vi "diffraction pattern v1.6.vi"() -> ()   [LabVIEW 2019]
panel:
  in  "Save":bool
  in  "hold":bool
  out "Current Flux":dbl=5.0
  out "Remaining steps":i32
  in  "Exit":bool
  in  "Run":bool
  out "Help":string="1. before run, set the paramaters on the left of the screen.\n2. flux (magnetic field) is in unit of flux quanta.\n3. Phaserange is in the unit of Pi, the CPR will be build up according to phase range of [-Phaserange/2,Phaserang/2], and such CPR will be  a periodic function with Phaserange as period. Enter integer number  of multiple times of 4 is preferred.\n4. Use the step setting tab to set resolution of the calculation, you can set how many points is used to define the width of the Josephson junction, how many points to represent the Phaserange\n5. Then you can choose which type of the CPR is used.\n6. Depending on the choose of the CPR, you may want to set the strength of the MBS, \"a\" parameter, the width of the gaussian function used, and the pattern of parity of MBS. Parity pattern has to have same number of elements for positive and negative range.\nEnter the parity 1 or -1 for positive and negative phase +-Pi, +-3Pi, +-5Pi etc.. in to the two arrays.\n7. You can use the index control to read the array elements, then enter the value, you can also delete an element of array by right click, the number of array elements is not limited.\n8. You can change the x,y range, zoom, create cursor etc. to help analyse the plot. Right click to save the data into excel.\n\nEnjoy!\nGuang Yue\n\n\n"
  in  "parity for negative phase":i32[](array[numeric])=[1, -1, -1, 1]
  in  "Strenth of MBS":dbl=0.5
  in  "parity for positive phase":i32[](array[numeric])=[1, -1, 1, 1]
  in  "Gaussian width":dbl=0.2
  in  "Tab Control":enum32{"Range", "Steps setting"}(tab)
  in  "flux start":dbl=-5.0
  in  "flux end":dbl=5.0
  in  "flux step":dbl=0.1
  in  "phaserange in Pi":i32=16
  in  "Geometry":i32=201
  in  "Phase steps":i32=201
  in  "CPR Type":T1(ring)
  out "Total time s":dbl=5.020437899999706
  in  "stop loop":bool
  out "Diffraction pattern plot":cluster{cluster{dbl, "icn":dbl}[]}[](graph)
  out "Ic negative":dbl=-0.0009989221220817583
  out "Ic positive":dbl=0.000998922122081775
  out "error out":errorcluster
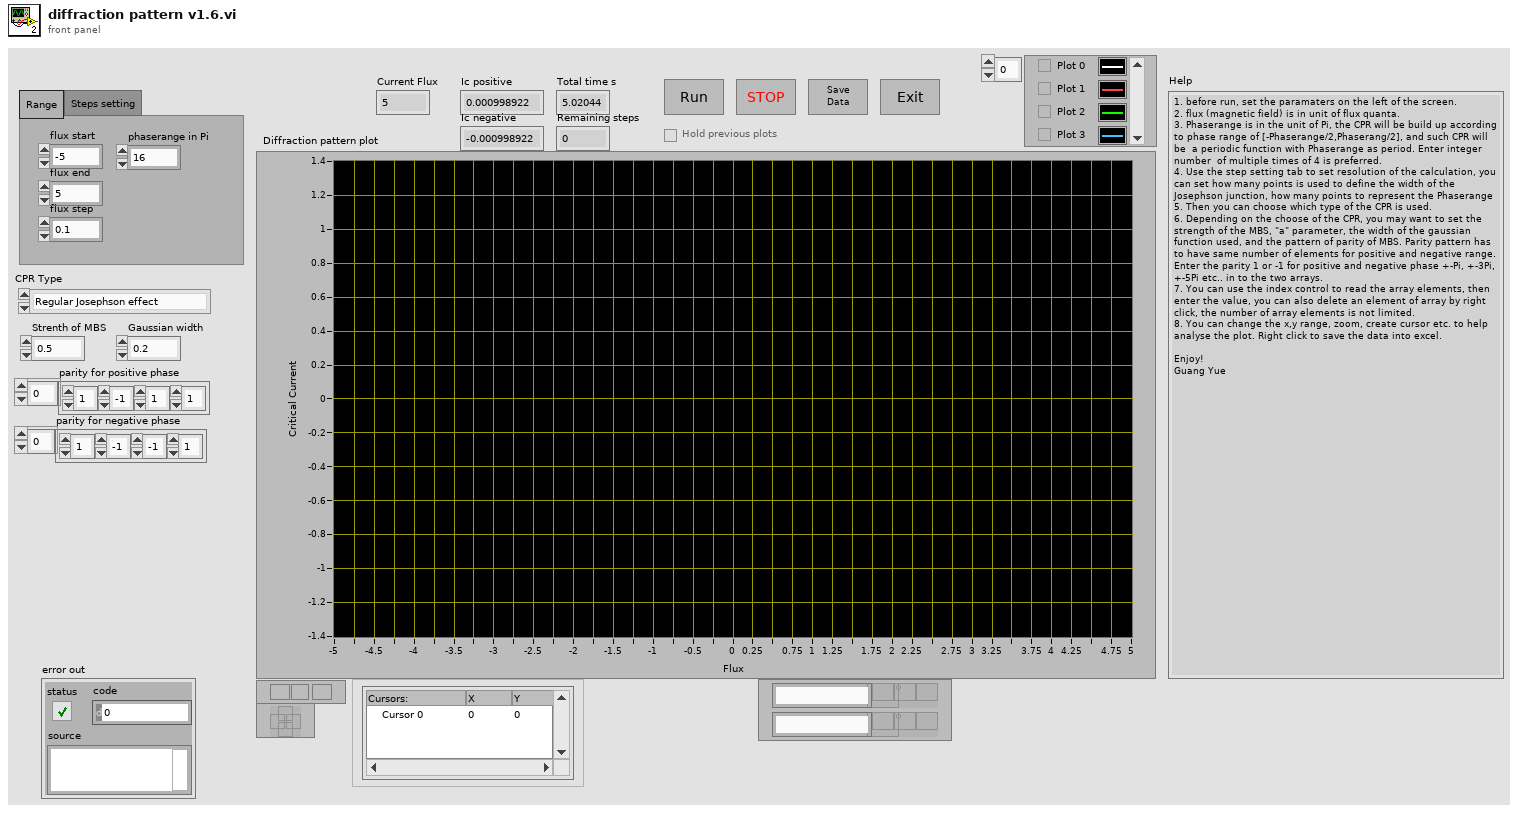
[diagram p1: front panel]
types:
  T1 = enum16{"Regular Josephson effect", "Non-local MBS", "Local MBS same parity", "Local MBS different parity"}
  T2 = enum32{"invalid app kind", "Development System", "Run Time System", "Student Edition", "Embedded LabVIEW", "Evaluation", "Custom"}
  T3 = enum8{"Enabled", "Disabled", "Disabled and Grayed Out"}
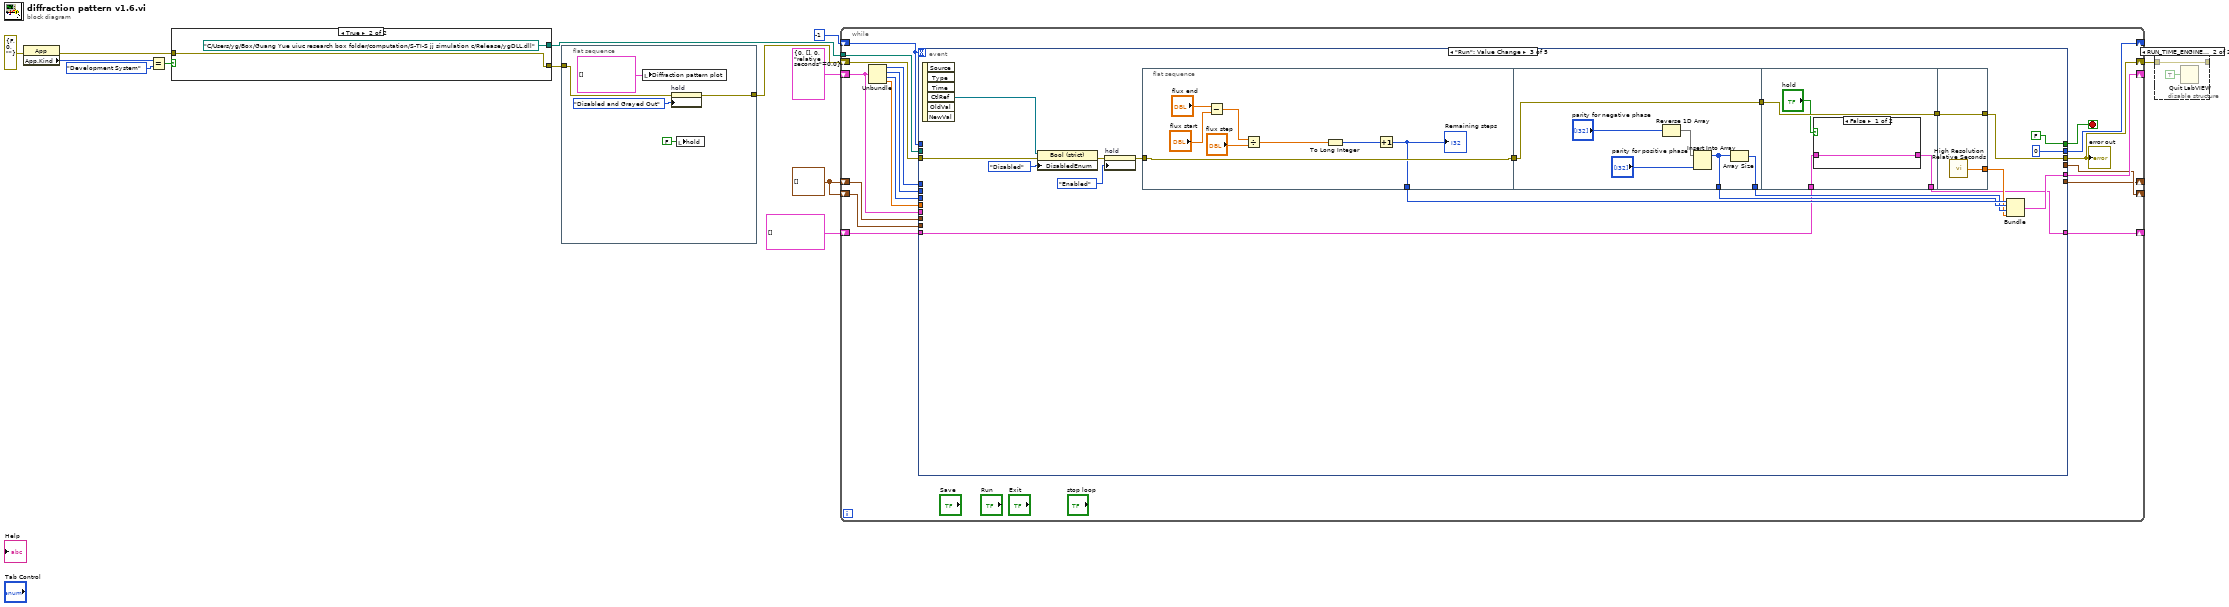
[diagram p0: block diagram]
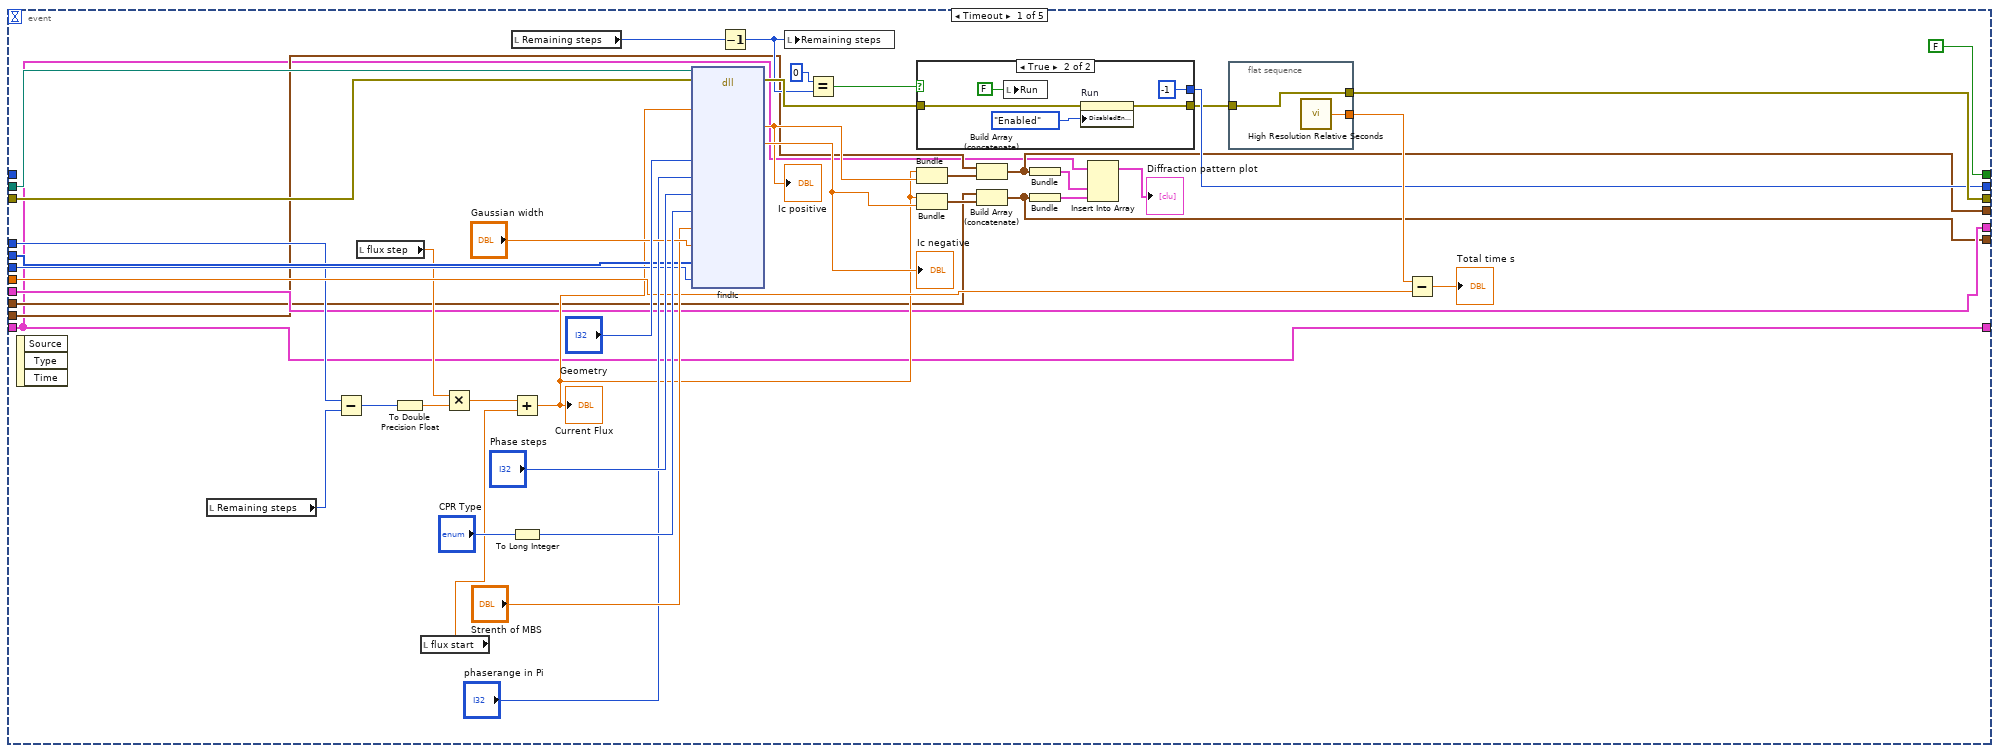
[diagram p3: hidden frame]
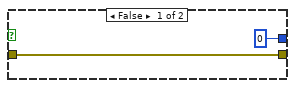
[diagram p4: hidden frame]
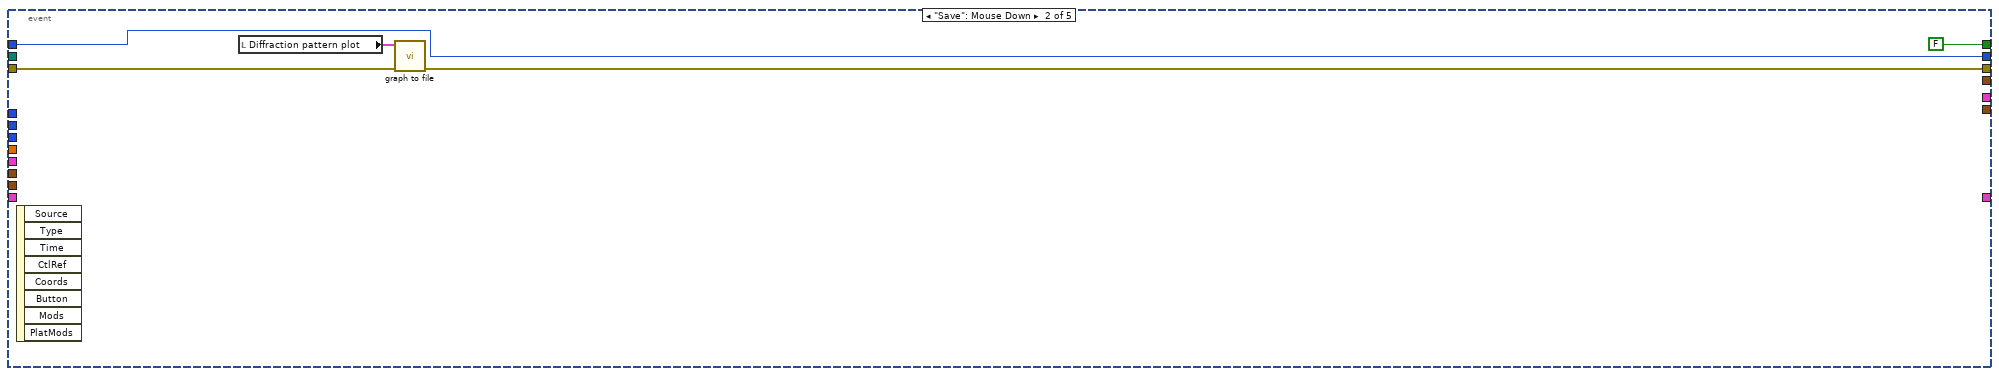
[diagram p5: hidden frame]
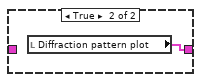
[diagram p6: hidden frame]
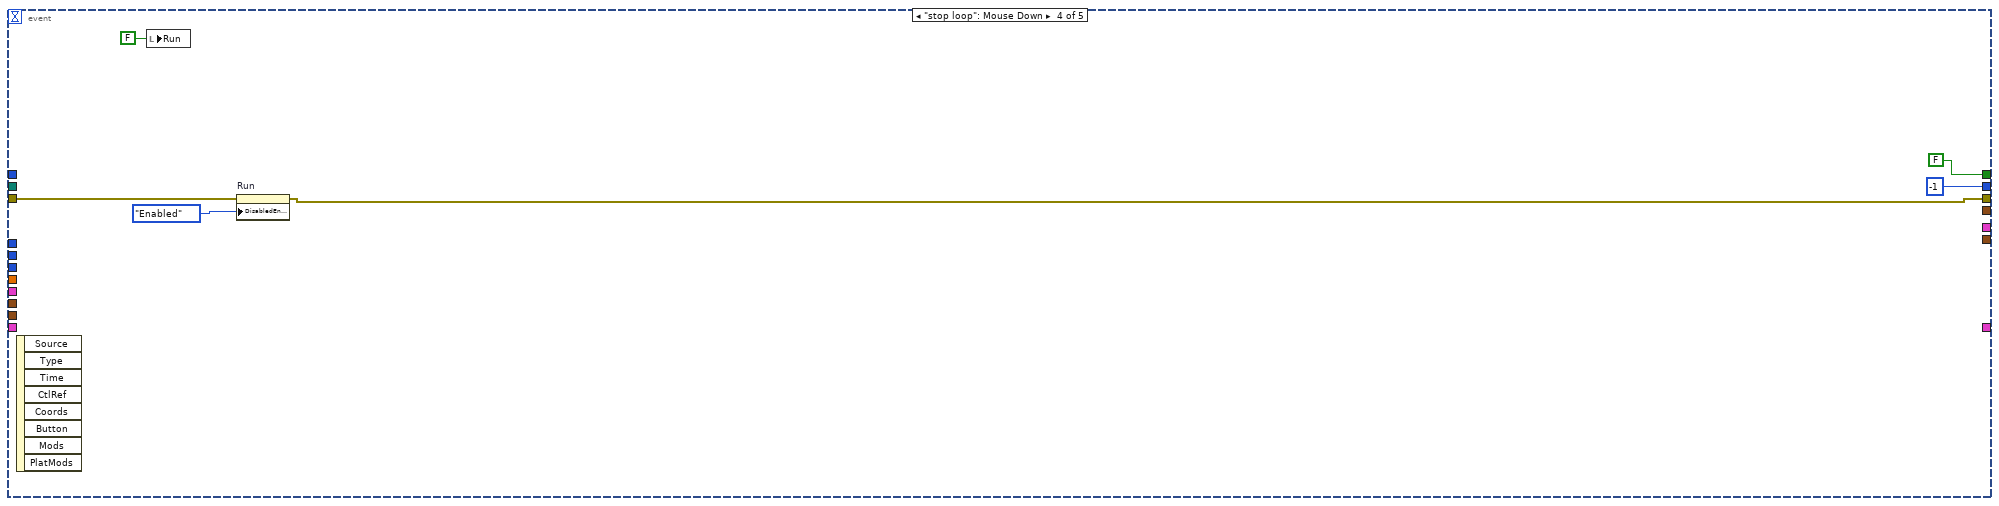
[diagram p7: hidden frame]
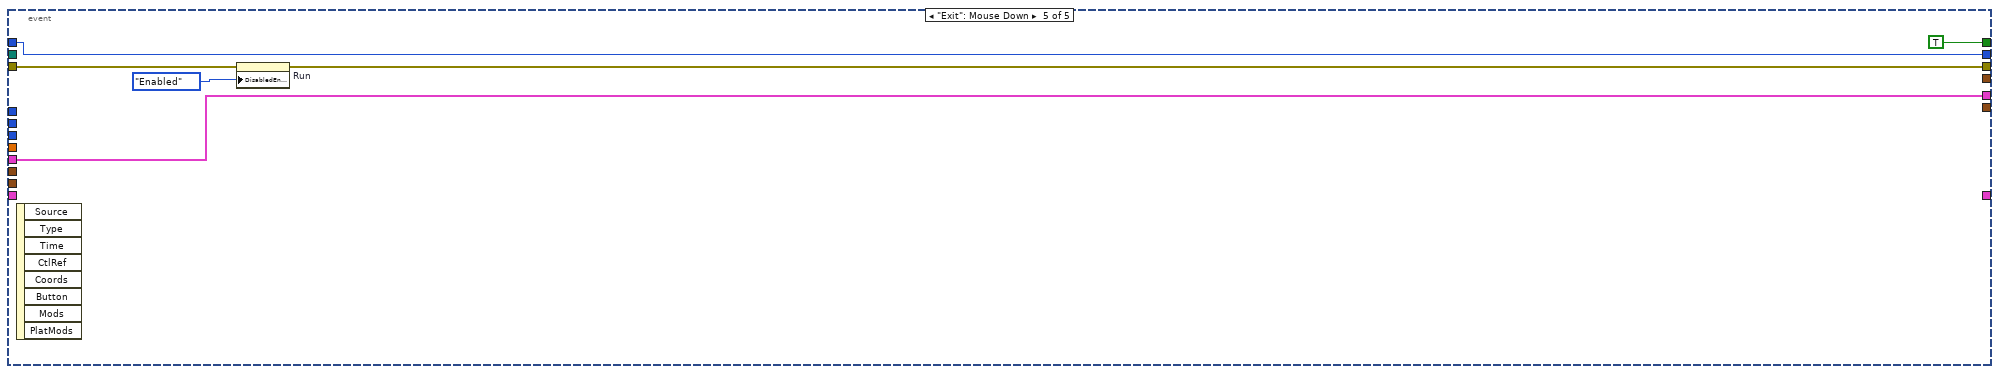
[diagram p8: hidden frame]
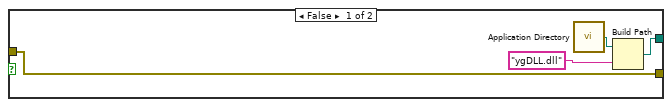
[diagram p9: hidden frame]
diagram:
  w5 = cluster{dbl, "inp":dbl}[] []
  n1 = property class="App"(error in=errorcluster {"status"=FALSE, "code"=0, "source"=""} ("error out")) -> (error out=w9:errorcluster, "App.Kind"=w12:T2)  [unwired: 1 in, 1 out]
  n2 = Equal?(x=w12, y=T2."Development System" ("Application:Kind")) -> (x = y?=w10:bool)
  n3 = case shown="True" w10 {
    tunnel: [w15 path "C:/Users/yg/Box/Guang Yue uiuc research box folder/computation/S-TI-S jj simulation c/Release/ygDLL.dll"] -> w8
    tunnel: w9 -> [w14 w18]
    tunnel: [w14 w18] -> w2
    frame False {
      n4 = call <vilib>:"Application Directory.vi"() -> ("Application Directory"=w17:path)
      n5 = Build Path(base path=w17, name or relative path="ygDLL.dll") -> (appended path=w15:path)
    }
    frame True {
    }
  }
  n6 = flat-sequence {
    tunnel: w2 -> [w23]
    tunnel: [w22] -> w1
    frame #0 {
      n7 = local write "Diffraction pattern plot"(cluster{cluster{dbl, "icn":dbl}[]}[] [] ("appended array")) -> ()
      n8 = property on="hold" class="Bool (strict)"(error in=w23, "DisabledEnum"=T3."Disabled and Grayed Out" ("Disabled")) -> (error out=w22:errorcluster)  [unwired: 1 in, 1 out]
      n9 = local write "hold"(FALSE ("hold")) -> ()
    }
  }
  n10 = while {
    tunnel: w8 -> [w39]
    shift-right: [w41] -> _
    shift-left: -1 -> [w32]
    shift-right: [w42] -> _
    shift-left: cluster{i32, i32[], i32, "relative seconds":dbl} {0, [], 0, "relative seconds"=0.0} -> [w33]
    shift-right: [w35] -> w4
    shift-left: w1 -> [w40]
    shift-right: [w30] -> _
    shift-left: w5 -> [w31]
    shift-right: [w29] -> _
    shift-left: w5 -> [w28]
    shift-right: [w25] -> _
    shift-left: cluster{cluster{dbl, "icn":dbl}[]}[] [] ("appended array") -> [w26]
    stop <- w27 stop-if-true
    n11 = Unbundle(w33) -> (w34:i32, w38:i32[], w37:i32, "relative seconds"=w36:dbl)
    n12 = event shown="[2] \"Run\": Value Change" {
      selector: _ -> [_ _ _ _ _]
      dyn-events: _ -> [_ _ _ _ _]
      timeout: w32 -> [_ _ _ _ _]
      tunnel: [w53 _ w112 _ w152] -> w42
      tunnel: [w55 w99 0 -1 w153] -> w41
      tunnel: w40 -> [w72 w98 w110 w146 w150]
      tunnel: w39 -> [w71 _ _ _ _]
      tunnel: w38 -> [w70 _ _ _ _]
      tunnel: w37 -> [w69 _ _ _ _]
      tunnel: w36 -> [w68 _ _ _ _]
      tunnel: [w67 w96 w109 w144 w148] -> w35
      tunnel: w34 -> [w66 _ _ _ _]
      tunnel: w33 -> [w53 _ _ _ w152]
      tunnel: w32 -> [_ w99 _ _ w153]
      tunnel: w31 -> [w50 _ _ _ _]
      tunnel: [w51 _ _ _ _] -> w30
      tunnel: [w49 _ _ _ _] -> w29
      tunnel: w28 -> [w48 _ _ _ _]
      tunnel: [FALSE FALSE FALSE FALSE TRUE] -> w27
      tunnel: w26 -> [w43 _ w104 _ _]
      tunnel: [w43 _ w105 _ _] -> w25
      event Timeout {
        n13 = event-data() -> ()  [unwired: 1 in, 3 out]
        n14 = local read "Remaining steps"() -> (w65:i32)
        n15 = Subtract(x=w66, y=w65) -> (x-y=w63:i32)
        n16 = local read "flux step"() -> (w64:dbl)
        n17 = To Double Precision Float(number=w63) -> (double precision float=w81:dbl)
        n18 = local read "flux start"() -> (w62:dbl)
        n19 = Multiply(x=w64, y=w81) -> (x*y=w82:dbl)
        n20 = local read "Remaining steps"() -> (w59:i32)
        n21 = Add(x=w82, y=w62) -> (x+y=w61:dbl)
        "Current Flux" <- w61
        n22 = To Long Integer(number="CPR Type") -> (32bit integer=w86:i32)
        n23 = dll-call lib="C:/Users/yg/Box/Guang Yue uiuc research box folder/computation/S-TI-S jj simulation c/Release/ygDLL.dll" fn="findIc"(path in=w71, error in=w72, "flux"=w61, "nw"="Geometry", "phaserange"="phaserange in Pi", "nphase"="Phase steps", "cpr"=w86, "a"="Strenth of MBS", "gw"="Gaussian width", "parity"=w70, "parity_l"=w69) -> (error out=w60:errorcluster, "inp"=w83:dbl, "icn"=w84:dbl)  [unwired: 13 in, 1 out]
        "Ic positive" <- w83
        "Ic negative" <- w84
        n24 = Decrement(x=w59) -> (x-1=w57:i32)
        n25 = local write "Remaining steps"(w57) -> ()
        n26 = Equal?(x=0, y=w57) -> (x = y?=w56:bool)
        n27 = case shown="True" w56 {
          tunnel: w60 -> [w87 w92]
          tunnel: [0 -1] -> w55
          tunnel: [w87 w91] -> w54
          frame False {
          }
          frame True {
            n28 = local write "Run"(FALSE ("Run")) -> ()
            n29 = property on="Run" class="Bool (strict)"(error in=w92, "DisabledEnum"=T3."Enabled" ("Disabled")) -> (error out=w91:errorcluster)  [unwired: 1 in, 1 out]
          }
        }
        n30 = Bundle(w61, "inp"=w83) -> (w52:cluster{dbl, "inp":dbl})  [unwired: 1 in]
        n31 = Bundle(w61, "icn"=w84) -> (w85:cluster{dbl, "icn":dbl})  [unwired: 1 in]
        n32 = Build Array (concatenate)(w50, w52) -> (w51:cluster{dbl, "inp":dbl}[])
        n33 = Build Array (concatenate)(w48, w85) -> (w49:cluster{dbl, "icn":dbl}[])
        n34 = Bundle(w51) -> (w46:cluster{cluster{dbl, "inp":dbl}[]})  [unwired: 1 in]
        n35 = Bundle(w49) -> (w45:cluster{cluster{dbl, "icn":dbl}[]})  [unwired: 1 in]
        n36 = Insert Into Array(array=w43, new element #1=w46, new element #2=w45) -> (→"Diffraction pattern plot":cluster{cluster{dbl, "icn":dbl}[]}[])  [unwired: 1 in]
        n37 = flat-sequence {
          tunnel: w54 -> [w95]
          tunnel: [w95] -> w67
          tunnel: [w94] -> w80
          frame #0 {
            n38 = call <vilib>:"High Resolution Relative Seconds.vi"() -> ("relative seconds"=w94:dbl)
          }
        }
        n39 = Subtract(x=w80, y=w68) -> (x-y=→"Total time s":dbl)
      }
      event "Save": Mouse Down {
        n40 = event-data() -> ()  [unwired: 1 in, 8 out]
        n41 = local read "Diffraction pattern plot"() -> (w97:cluster{cluster{dbl, "icn":dbl}[]}[])
        n42 = call "graph to file.vi"("error in (no error)"=w98, "Input array"=w97) -> ("error out"=w96:errorcluster)  [unwired: 9 in]
      }
      event "Run": Value Change {
        n43 = event-data() -> ("CtlRef"=w119:refnum<vi>)  [unwired: 1 in, 5 out]
        n44 = property class="Bool (strict)"(reference=w119, error in=w110, "DisabledEnum"=T3."Disabled" ("Disabled")) -> (error out=w103:errorcluster)  [unwired: 1 out]
        n45 = property on="hold" class="Bool (strict)"(error in=w103, "DisabledEnum"=T3."Enabled" ("Disabled")) -> (error out=w102:errorcluster)  [unwired: 1 in, 1 out]
        n46 = flat-sequence {
          tunnel: w102 -> [w121]
          tunnel: [w120] -> w116
          tunnel: [w121] -> w117
          tunnel: w117 -> [w133]
          tunnel: [w129] -> w114
          tunnel: [w128] -> w115
          tunnel: [w133] -> w107
          tunnel: w107 -> [w137]
          tunnel: [w137] -> w106
          tunnel: [w135] -> w105
          tunnel: w104 -> [w134]
          tunnel: [w141] -> w109
          tunnel: w106 -> [w141]
          tunnel: [w140] -> w113
          frame #0 {
            n47 = Subtract(x="flux end", y="flux start") -> (x-y=w126:dbl)
            n48 = Divide(x=w126, y="flux step") -> (x/y=w125:dbl)
            n49 = To Long Integer(number=w125) -> (32bit integer=w124:i32)
            n50 = Increment(x=w124) -> (x+1=w120:i32)
            "Remaining steps" <- w120
          }
          frame #1 {
            n51 = Reverse 1D Array(array="parity for negative phase") -> (reversed array=w131:i32[])
            n52 = Insert Into Array(array=w131, new element="parity for positive phase") -> (w128:i32[])  [unwired: 1 in]
            n53 = Array Size(array=w128) -> (size(s)=w129:i32)
          }
          frame #2 {
            n54 = case shown="False" "hold" {
              tunnel: [w138 w139] -> w135
              tunnel: w134 -> [w138 _]
              frame False {
              }
              frame True {
                n55 = local read "Diffraction pattern plot"() -> (w139:cluster{cluster{dbl, "icn":dbl}[]}[])
              }
            }
          }
          frame #3 {
            n56 = call <vilib>:"High Resolution Relative Seconds.vi"() -> ("relative seconds"=w140:dbl)
          }
        }
        n57 = Bundle(w116, w115, w114, "relative seconds"=w113) -> (w112:cluster{i32, i32[], i32, "relative seconds":dbl})  [unwired: 1 in]
      }
      event "stop loop": Mouse Down {
        n58 = event-data() -> ()  [unwired: 1 in, 8 out]
        n59 = local write "Run"(FALSE ("Run")) -> ()
        n60 = property on="Run" class="Bool (strict)"(error in=w146, "DisabledEnum"=T3."Enabled" ("Disabled")) -> (error out=w144:errorcluster)  [unwired: 1 in, 1 out]
      }
      event "Exit": Mouse Down {
        n61 = event-data() -> ()  [unwired: 1 in, 8 out]
        n62 = property on="Run" class="Bool (strict)"(error in=w150, "DisabledEnum"=T3."Enabled" ("Disabled")) -> (error out=w148:errorcluster)  [unwired: 1 in, 1 out]
      }
    }
    "error out" <- w35
  }
  n63 = disable-structure shown="RUN_TIME_ENGINE==True" {
    disable-tunnel: [w154 w155] -> _
    disable-tunnel: w4 -> [w154 w155]
    frame condition #0 (active) {
    }
    frame condition #1 {
      n64 = Quit LabVIEW(quit? (T)=TRUE) -> ()
    }
  }
